vi "Swerve Go To.vi"(0 "Max Speed":dbl, 1 "Target X":dbl, 2 "Target Y":dbl, 3 "Target Angle":dbl) -> (6 "Done":bool)   [LabVIEW 2016, in "CAN Talon SRX Swerve.lvlib"]
uses:
  CAN Talon SRX Swerve.lvlib
  <vilib>/addons/control/pid/pid.llb/PID (DBL).vi
  <vilib>/addons/control/pid/NI_PID_pid.lvlib
  Apple Gyro/Apple Pi Gyro Library.lvlib
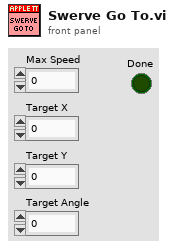
[diagram p1: front panel]
types:
  T1 = enum16{"Prepare to Rotate", "Rotate", "Prepare to Move", "Move"}
  T2 = cluster{"proportional gain (Kc)":dbl, "integral time (Ti, min)":dbl, "derivative time (Td, min)":dbl}
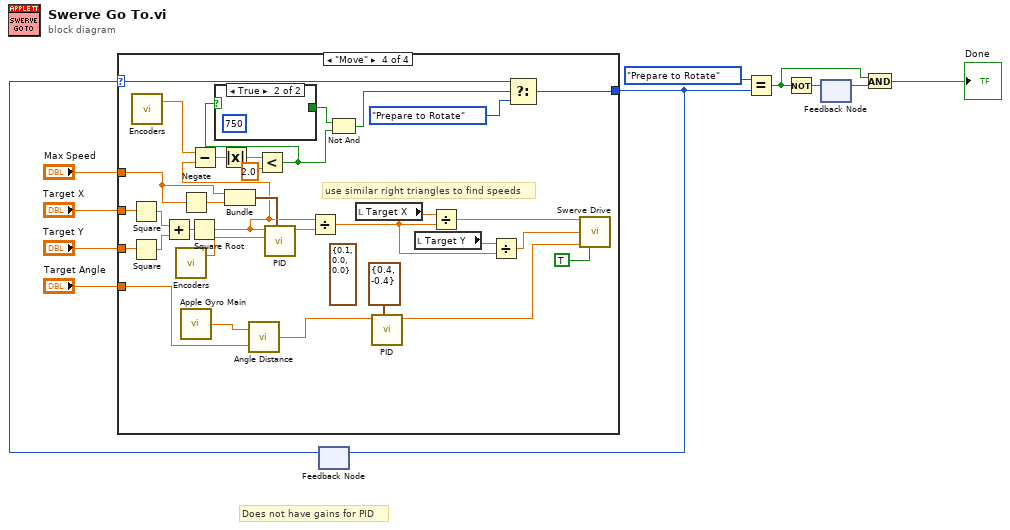
[diagram p0: block diagram]
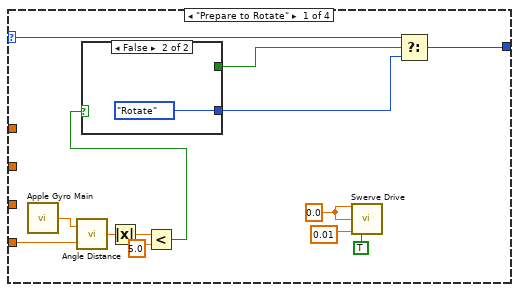
[diagram p2: hidden frame]
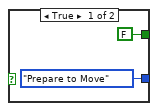
[diagram p3: hidden frame]
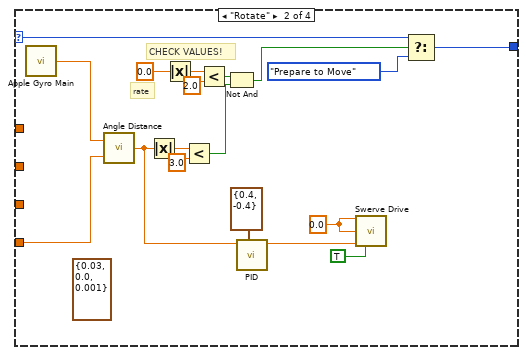
[diagram p4: hidden frame]
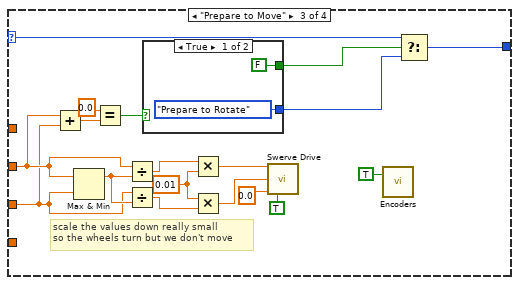
[diagram p5: hidden frame]
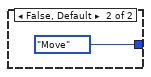
[diagram p6: hidden frame]
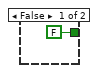
[diagram p7: hidden frame]
diagram:
  # "Does not have gains for PID"
  n1 = feedback #1() -> (w6:T1)  [unwired: 1 in]
  n2 = case shown="\"Move\"" w6 {
    selector: w6 -> [w23 w44 w62 w97]
    tunnel: [w24 w45 w63 w98] -> w1
    tunnel: "Target Angle" -> [w20 w32 _ w80]
    tunnel: "Target X" -> [_ _ w54 w95]
    tunnel: "Target Y" -> [_ _ w53 w94]
    tunnel: "Max Speed" -> [_ _ _ w88]
    frame "Prepare to Rotate" {
      w22 = 0.0
      n3 = call "Apple Gyro Main.vi"() -> ("Gyro Yaw Out"=w12:dbl)  [unwired: 4 in]
      n4 = call "Angle Distance.vi"("target angle"=w20, "current angle"=w12) -> ("distance"=w19:dbl)
      n5 = Absolute Value(x=w19) -> (abs(x)=w18:dbl)
      n6 = Less?(x=w18, y=5.0) -> (x < y?=w16:bool)
      n7 = case shown="False" w16 {
        tunnel: [FALSE _] -> w14
        tunnel: [T1."Prepare to Move" T1."Rotate"] -> w15
        frame True {
        }
        frame False, Default {
        }
      }
      n8 = call "Swerve Drive.vi"("X"=w22, "Y"=w22, "Z"=0.01, "Auto Controls"=TRUE) -> ()  [unwired: 11 in, 1 out]
      n9 = Select(t=w23, s=w14, f=w15) -> (s? t:f=w24:T1)
    }
    frame "Rotate" {
      (unwired) T2 {"proportional gain (Kc)"=0.03, "integral time (Ti, min)"=0.0, "derivative time (Td, min)"=0.001} ("PID gains")
      w42 = 0.0
      # "rate"
      # "CHECK VALUES!"
      n10 = call "Apple Gyro Main.vi"() -> ("Gyro Yaw Out"=w29:dbl)  [unwired: 4 in]
      n11 = call "Angle Distance.vi"("target angle"=w32, "current angle"=w29) -> ("distance"=w31:dbl)
      n12 = Absolute Value(x=w31) -> (abs(x)=w37:dbl)
      n13 = Absolute Value(x=0.0) -> (abs(x)=w40:dbl)
      n14 = Less?(x=w37, y=3.0) -> (x < y?=w34:bool)
      n15 = Less?(x=w40, y=2.0) -> (x < y?=w36:bool)
      n16 = Not And(1:w34, 2:w36) -> (0:w35:bool)
      n17 = call-poly <vilib>:"PID.vi"("output range"=cluster{"output high":dbl, "output low":dbl} {"output high"=0.4, "output low"=-0.4}, "setpoint"=w31) -> ("output"=w33:dbl)  [unwired: 8 in, 1 out]
      n18 = call "Swerve Drive.vi"("X"=w42, "Y"=w42, "Z"=w33, "Auto Controls"=TRUE) -> ()  [unwired: 11 in, 1 out]
      n19 = Select(t=w44, s=w35, f=T1."Prepare to Move") -> (s? t:f=w45:T1)
    }
    frame "Prepare to Move" {
      w60 = 0.01 ("y")
      # "scale the values down really small\nso the wheels turn but we don't move"
      n20 = Add(x=w54, y=w53) -> (x+y=w52:dbl)
      n21 = Max & Min(x=w54, y=w53) -> (max(x,y)=w61:dbl)  [unwired: 1 out]
      n22 = Equal?(x=0.0, y=w52) -> (x = y?=w50:bool)
      n23 = Divide(x=w54, y=w61) -> (x/y=w58:dbl)
      n24 = Divide(x=w53, y=w61) -> (x/y=w59:dbl)
      n25 = case shown="True" w50 {
        tunnel: [FALSE _] -> w48
        tunnel: [T1."Prepare to Rotate" T1."Move"] -> w49
        frame True {
        }
        frame False, Default {
        }
      }
      n26 = Multiply(x=w58, y=w60) -> (x*y=w57:dbl)
      n27 = Multiply(x=w60, y=w59) -> (x*y=w56:dbl)
      n28 = call "Swerve Drive.vi"("X"=w57, "Y"=w56, "Z"=0.0, "Auto Controls"=TRUE) -> ()  [unwired: 11 in, 1 out]
      n29 = call "Encoders.vi"("Reset All"=TRUE) -> ()  [unwired: 1 in, 2 out]
      n30 = Select(t=w62, s=w48, f=w49) -> (s? t:f=w63:T1)
    }
    frame "Move" {
      (unwired) T2 {"proportional gain (Kc)"=0.1, "integral time (Ti, min)"=0.0, "derivative time (Td, min)"=0.0} ("PID gains")
      # "use similar right triangles to find speeds"
      n31 = Square(x=w95) -> (x^2=w93:dbl)
      n32 = Square(x=w94) -> (x^2=w92:dbl)
      n33 = call "Encoders.vi"() -> ("Avg Absolute Distance"=w77:dbl)  [unwired: 2 in, 1 out]
      n34 = Add(x=w93, y=w92) -> (x+y=w91:dbl)
      n35 = call "Encoders.vi"() -> ("Avg Absolute Distance"=w81:dbl)  [unwired: 2 in, 1 out]
      n36 = Negate(x=w88) -> (-x=w89:dbl)
      n37 = call "Apple Gyro Main.vi"() -> ("Gyro Yaw Out"=w76:dbl)  [unwired: 4 in]
      n38 = Square Root(x=w91) -> (sqrt(x)=w74:dbl)
      n39 = Subtract(x=w77, y=w74) -> (x-y=w85:dbl)
      n40 = Absolute Value(x=w85) -> (abs(x)=w86:dbl)
      n41 = Bundle("Max Speed"=w88, w89) -> (w90:cluster{"Max Speed":dbl, dbl})  [unwired: 1 in]
      n42 = call "Angle Distance.vi"("target angle"=w80, "current angle"=w76) -> ("distance"=w79:dbl)
      n43 = Less?(x=w86, y=2.0) -> (x < y?=w67:bool)
      n44 = case shown="True" w67 {
        tunnel: [FALSE _] -> w68
        frame False {
        }
        frame True {
          (unwired) 750 ("Time (ms)")
        }
      }
      n45 = call-poly <vilib>:"PID.vi"("output range"=w90, "process variable"=w81, "setpoint"=w74) -> ("output"=w75:dbl)  [unwired: 7 in, 1 out]
      n46 = Divide(x=w74, y=w75) -> (x/y=w72:dbl)
      n47 = Not And(1:w67, 2:w68) -> (0:w84:bool)
      n48 = local read "Target X"() -> (w73:dbl)
      n49 = call-poly <vilib>:"PID.vi"("output range"=cluster{"output high":dbl, "output low":dbl} {"output high"=0.4, "output low"=-0.4}, "setpoint"=w79) -> ("output"=w82:dbl)  [unwired: 8 in, 1 out]
      n50 = local read "Target Y"() -> (w71:dbl)
      n51 = Divide(x=w73, y=w72) -> (x/y=w69:dbl)
      n52 = Divide(x=w71, y=w72) -> (x/y=w70:dbl)
      n53 = Select(t=w97, s=w84, f=T1."Prepare to Rotate") -> (s? t:f=w98:T1)
      n54 = call "Swerve Drive.vi"("X"=w69, "Y"=w70, "Z"=w82, "Auto Controls"=TRUE) -> ()  [unwired: 11 in, 1 out]
    }
  }
  n55 = feedback-in #1(w1) -> ()
  n56 = Equal?(x=T1."Prepare to Rotate", y=w1) -> (x = y?=w2:bool)
  n57 = Not(x=w2) -> (.not. x?=w4:bool)
  n58 = feedback #2() -> (w3:bool)  [unwired: 1 in]
  n59 = feedback-in #2(w4) -> ()
  n60 = And(x=w2, y=w3) -> (x .and. y?=→"Done":bool)
